vi "GetParam.vi"(8 "error in (no error)":errorcluster caption="entrée d'erreur (pas d'erreur)", 11 "Adjusted_Mutual_Info_Score.lvclass":refnum<class "Adjusted_Mutual_Info_Score.lvclass">) -> (0 "error out":errorcluster caption="sortie d'erreur", 2 "adjusted_mutual_info_score":cluster{"average_method":string}={"average_method"="arithmetic"}, 3 "Adjusted_Mutual_Info_Score.lvclass":refnum<class "Adjusted_Mutual_Info_Score.lvclass">)   [LabVIEW 2020, in "Adjusted_Mutual_Info_Score.lvclass"]
doc: "Get Parameters"
uses:
  Adjusted_Mutual_Info_Score.lvclass
  Adjusted_Mutual_Info_Score.lvclass/Adjusted_Mutual_Info_Score.ctl
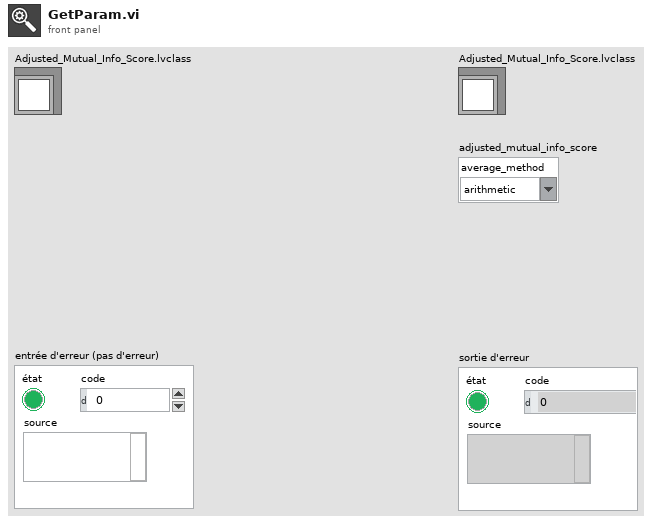
[diagram p1: front panel]
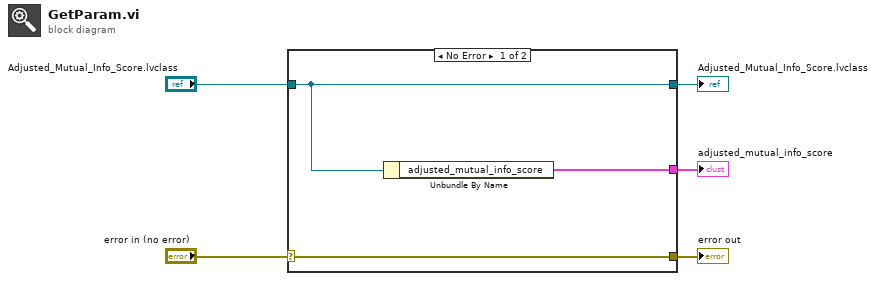
[diagram p0: block diagram]
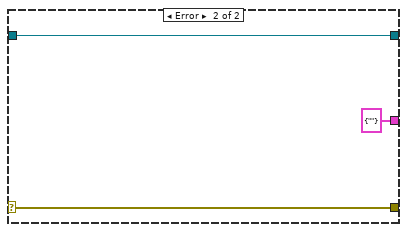
[diagram p2: hidden frame]
diagram:
  n1 = case shown="No Error" "error in (no error)" {
    selector: "error in (no error)" -> [w8 w10]
    tunnel: [w8 w10] -> w4
    tunnel: [w7 w11] -> w2
    tunnel: "Adjusted_Mutual_Info_Score.lvclass" -> [w7 w11]
    tunnel: [w6 cluster{"average_method":string} {"average_method"=""} ("adjusted_mutual_info_score")] -> w1
    frame No Error {
      n2 = Unbundle By Name(w7) -> ("adjusted_mutual_info_score"=w6:cluster{"average_method":string})
    }
    frame Error {
    }
  }
  "error out" <- w4
  "Adjusted_Mutual_Info_Score.lvclass" <- w2
  "adjusted_mutual_info_score" <- w1
